vi "FTW-Actor-Core-Initialize.vi"(0 "FTW Actor Instance":refnum<class "FTW-Actor-Instance.lvclass">, 5 "Inbox Configuration":string, 7 "Primary Inbox Address":string, 9 "Supervisor Address":string, 11 "error in":errorcluster) -> (4 "FTW Actor Instance out":refnum<class "FTW-Actor-Instance.lvclass">, 6 "Incoming Request":refnum<event-registration>, 8 "Resolved Primary Inbox Address":string, 15 "error out":errorcluster)   [LabVIEW 2014, in "FTW-Actor-Instance.lvclass"]
uses:
  FTW-Actor-Instance.lvclass
  json/core/FTW-JSON-Core-Structure.ctl
  FTW-Actor-Instance.lvclass/FTW-Actor-Instance.ctl
  supervisor/connector/FTW-Supervisor-Connector.lvclass
panel:
  # "Inputs"
  # "Outputs"
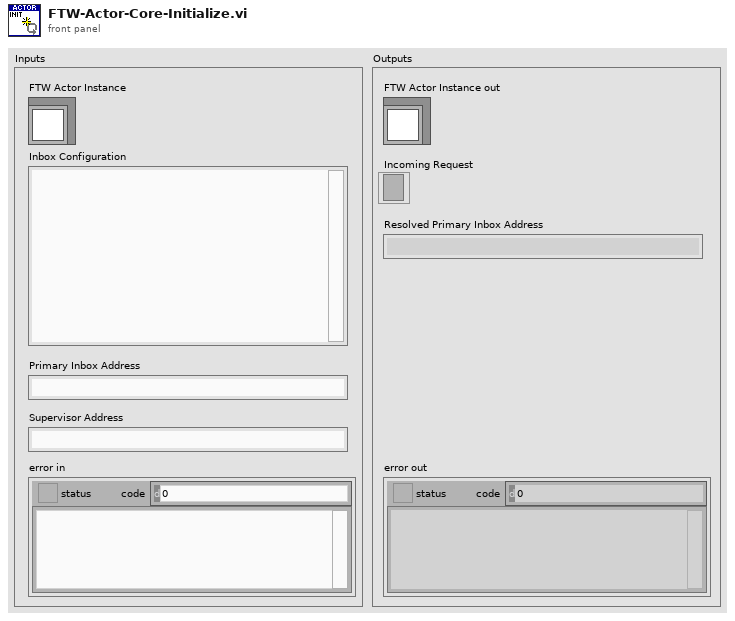
[diagram p1: front panel]
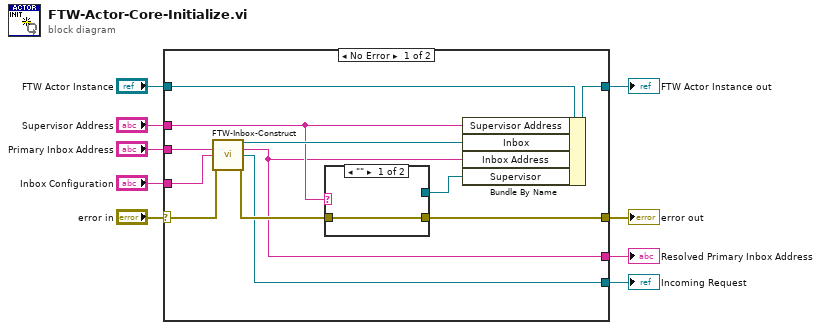
[diagram p0: block diagram]
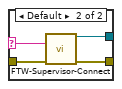
[diagram p2: hidden frame]
diagram:
  n1 = case shown="No Error" "error in" {
    selector: "error in" -> [w15 w27]
    tunnel: "FTW Actor Instance" -> [w21 w28]
    tunnel: [w10 _] -> w8
    tunnel: [w20 w28] -> w7
    tunnel: "Supervisor Address" -> [w16 _]
    tunnel: [w14 w27] -> w4
    tunnel: "Inbox Configuration" -> [w13 _]
    tunnel: [w11 _] -> w2
    tunnel: "Primary Inbox Address" -> [w12 _]
    frame No Error {
      n2 = call "FTW-Inbox-Construct.vi"("Primary Inbox Address"=w12, "Inbox Configuration"=w13, "error in"=w15) -> ("FTW Router"=w19:refnum<data-value>, "Resolved Primary Inbox Address"=w11:string, "Incoming Request"=w10:refnum<event-registration>, "error out"=w18:errorcluster)  [unwired: 9 in]
      n3 = case shown="\"\"" w16 {
        selector: w16 -> [_ w23]
        tunnel: [w22 w26] -> w14
        tunnel: w18 -> [w22 w25]
        tunnel: [_ w24] -> w17
        frame "" {
        }
        frame Default {
          n4 = call "FTW-Supervisor-Connect.vi"("Supervisor Address"=w23, "error in"=w25) -> ("FTW Supervisor Connection"=w24:refnum<class "FTW-Supervisor-Connector.lvclass">, "error out"=w26:errorcluster)  [unwired: 12 in]
        }
      }
      n5 = Bundle By Name(cluster=w21, "Supervisor Address"=w16, "Inbox"=w19, "Inbox Address"=w11, "Supervisor"=w17) -> (w20:refnum<class "FTW-Actor-Instance.lvclass">)
    }
    frame Error {
    }
  }
  "FTW Actor Instance out" <- w7
  "error out" <- w4
  "Incoming Request" <- w8
  "Resolved Primary Inbox Address" <- w2
